vi "anglecorrecting.vi"(11 "Current angle":dbl) -> (3 "Corrected angle":dbl)   [LabVIEW 2012]
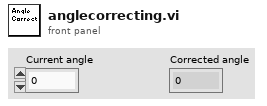
[diagram p1: front panel]
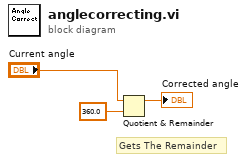
[diagram p0: block diagram]
diagram:
  # "Gets The Remainder"
  n1 = Quotient & Remainder(x="Current angle", y=360.0) -> (x-y*floor(x/y)=→"Corrected angle":dbl)  [unwired: 1 out]
